vi "TCP global names.vi"() -> ()   [LabVIEW 2015, in "TCP.lvlib"]
uses:
  TCP.lvlib
panel:
  out "Connected with client":string="Connected with client"
  out "Disconnected with":string="Disconnected with "
  out "Message sent to":string="Message sent to "
  out "No connection - data not sent!":string="No connection - data not sent!"
  out "Connection stopped":string="Connection stopped"
  out "Message received from":string="Message received from "
  out "No connection with":string="No connection with "
  out "Client mode. Opening connection...":string="Client mode. Connecting..."
  out "Connected with":string="Connected with "
  out "Server mode. Listening...":string="Server mode. Listening..."
  # "TCP messages"
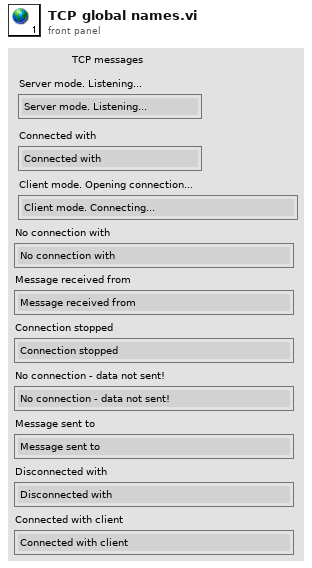
[diagram p1: front panel]
diagram:
